vi "session_handshake.vi"() -> ()   [LabVIEW 2013, in "libssh2_integration_tests.lvlib"]
uses:
  libssh2_integration_tests.lvlib
  <vilib>/addons/_JKI Toolkits/Caraya/classes/Assert/Assert Not Error.vi
  <vilib>/addons/_JKI Toolkits/Caraya/classes/Test/Test.lvclass
  <vilib>/addons/_JKI Toolkits/Caraya/classes/Assert/Assert.lvclass
panel:
  out "error out":errorcluster
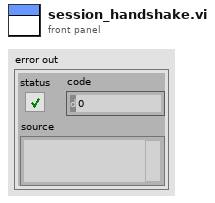
[diagram p1: front panel]
types:
  T1 = typedef "libssh2.lvlib/Session Refnum.ctl" = refnum<k1>
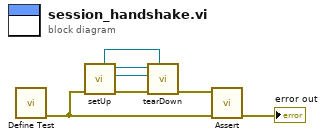
[diagram p0: block diagram]
diagram:
  n1 = call <vilib>:"Define Test.vi"() -> ("error out"=w6:errorcluster)  [unwired: 10 in, 1 out]
  n2 = call "setUp.vi"("error in (no error)"=w6) -> ("error out"=w5:errorcluster, "connection ID"=w4:refnum<k5>, "session"=w3:T1, "fixture"=w2:refnum<class "Server Fixture.lvclass">)  [unwired: 7 in]
  n3 = call "tearDown.vi"("fixture"=w2, "error in (no error)"=w5, "connection ID"=w4, "session"=w3) -> ("error out"=w1:errorcluster)  [unwired: 7 in]
  n4 = call-poly <vilib>:"Assert.vi"("error in (no error)"=w6, "Not Error?"=w1) -> ("error out"=→"error out":errorcluster)  [unwired: 8 in, 1 out]
